vi "smsAt (SubVI).vi"() -> ()   [LabVIEW 2012]
doc: "Demonstrates general use of Obtain Queue, queues and the effects different settings have on queue behavior. It uses a queue to pass data between an Enqueue loop (producing data) and a Dequeue loop (consuming data). If both loops run at the same speed, the queue does not fill up.\n\nWhen the Enqueue loop runs fast and the Dequeue loop runs slow, the queue quickly fills up and the Enqueue loop must wait for the Dequeue loop to remove elements. If the Enqueue loop runs slow and the Dequeue loop runs fast, the queue is quickly emptied and the Dequeue loop must wait for the Enqueue loop to insert elements."
uses:
  <vilib>/Instr/_visa.llb/VISA Set IO Buffer Mask.ctl
  <vilib>/Instr/_visa.llb/VISA Configure Serial Port (Instr).vi
panel:
  out "num":string
  out "read buffer":string
  out "Serial Settings:Data Bits":u16
  in  "VISA resource name":refnum<visa-resource-name>="COM4"
  out "last SMS":string
  out "Elements in Queue":i32
  in  "stop":bool
  in  "Queue Size":i32=50
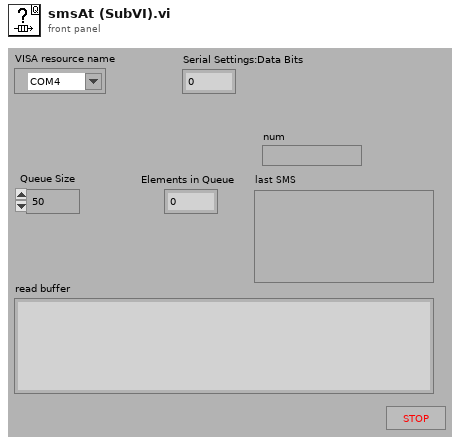
[diagram p1: front panel]
types:
  T1 = typedef "VISA Set IO Buffer Mask.ctl" = u16
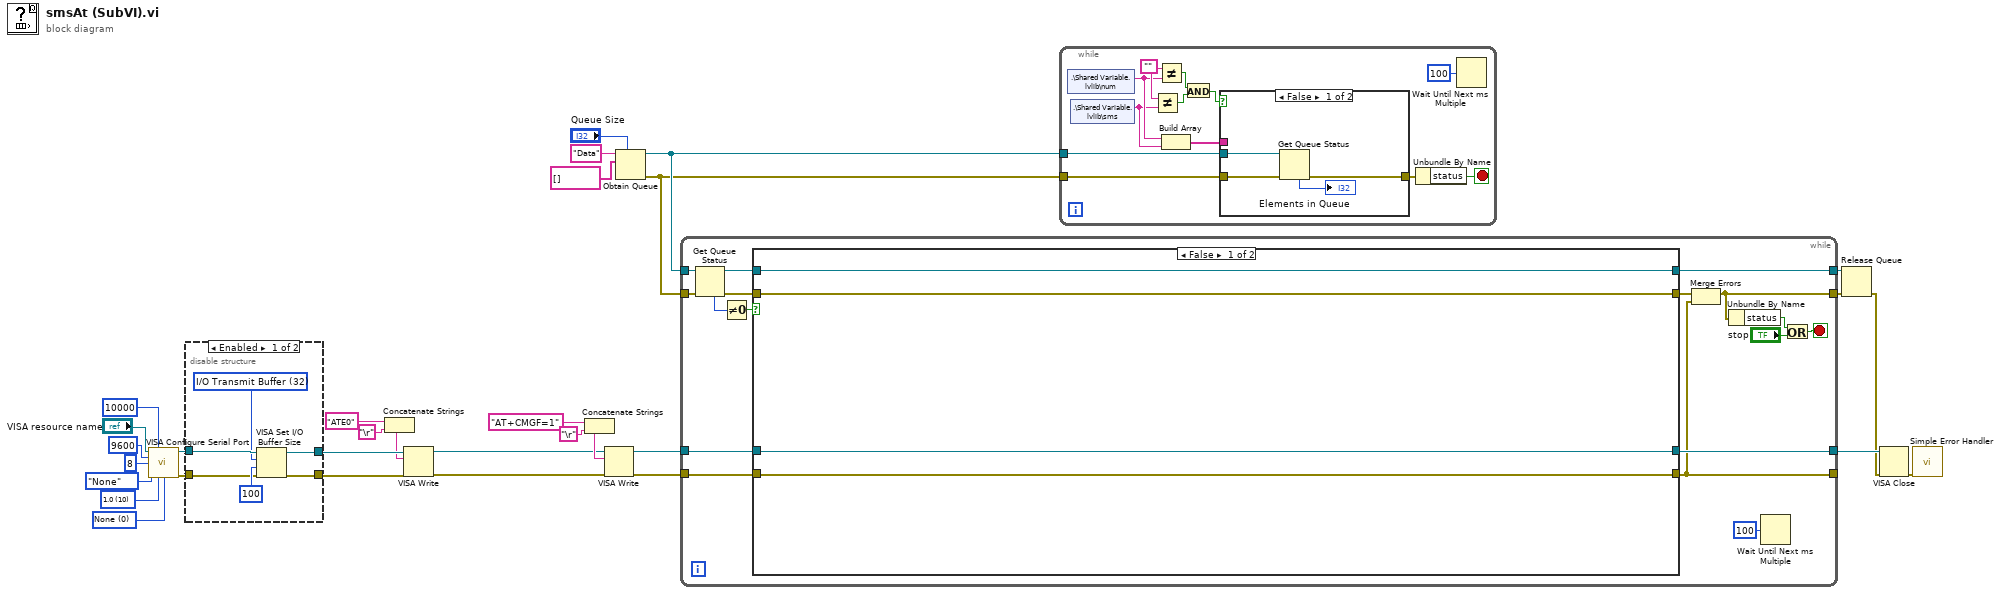
[diagram p0: block diagram]
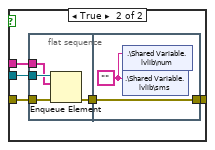
[diagram p3: hidden frame]
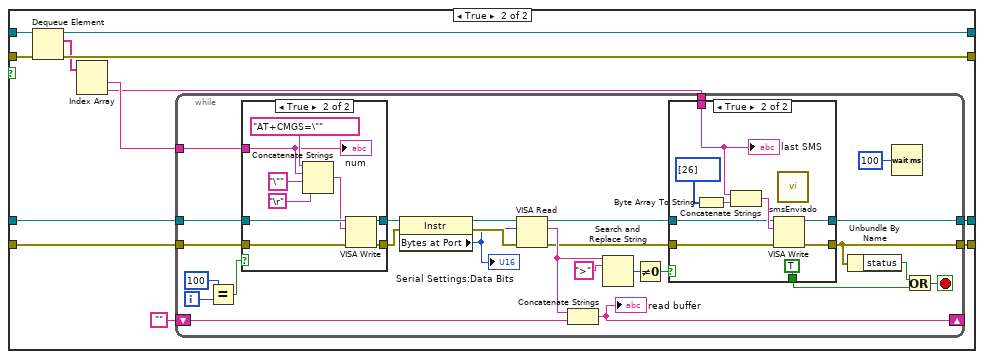
[diagram p4: hidden frame]
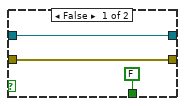
[diagram p5: hidden frame]
diagram:
  w22 = u16 0 items=["None", "XON/XOFF", "RTS/CTS", "XON/XOFF & RTS/CTS", "DTR/DSR", "XON/XOFF & DTR/DSR"] ("flow control (0:none)")
  w26 = u16 10 items=["1.0"=10, "1.5"=15, "2.0"=20] ("stop bits (10: 1 bit)")
  n1 = call-poly "VISA Configure Serial Port"("VISA resource name"="VISA resource name", "timeout (10sec)"=u32 10000, "baud rate (9600)"=u32 9600, "data bits (8)"=u16 8, "parity (0:none)"=enum16{"None", "Odd", "Even", "Mark", "Space"}."None", "stop bits (10: 1 bit)"=w26, "flow control (0:none)"=w22) -> ("VISA resource name out"=w20:refnum<visa-resource-name>, "error out"=w14:errorcluster)  [unwired: 7 in]
  n2 = disable-structure shown="Enabled" {
    disable-tunnel: w20 -> [w37 w39]
    disable-tunnel: [w34 w39] -> w19
    disable-tunnel: [w33 w38] -> w18
    disable-tunnel: w14 -> [w32 w38]
    frame Enabled {
      w35 = T1 32 items=["I/O Receive Buffer"=16, "I/O Transmit Buffer"=32, "I/O Receive and Transmit Buffer"=48] ("Mask")
      n3 = VISA Set I/O Buffer Size(VISA resource name=w37, mask (16)=w35, size (4096)=u32 100, error in (no error)=w32) -> (VISA resource name out=w34:refnum<visa-resource-name>, error out=w33:errorcluster)
    }
    frame Disabled {
    }
  }
  n4 = Concatenate Strings("ATE0" ("write buffer"), "\r") -> (w15:string)
  n5 = VISA Write(VISA resource name=w19, write buffer=w15, error in (no error)=w18) -> (VISA resource name out=w3:refnum<visa-resource-name>, error out=w4:errorcluster)  [unwired: 1 out]
  n6 = Concatenate Strings("AT+CMGF=1" ("write buffer"), "\r") -> (w7:string)
  n7 = VISA Write(VISA resource name=w3, write buffer=w7, error in (no error)=w4) -> (VISA resource name out=w2:refnum<visa-resource-name>, error out=w1:errorcluster)  [unwired: 1 out]
  n8 = Obtain Queue(max queue size (-1, unlimited)="Queue Size", name (unnamed)="Data", element data type=string[] []) -> (queue out=w31:refnum<queue>, error out=w29:errorcluster)  [unwired: 2 in, 1 out]
  n9 = while {
    tunnel: w31 -> [w56]
    tunnel: w29 -> [w52]
    tunnel: [w47] -> w28
    tunnel: w2 -> [w45]
    tunnel: w1 -> [w46]
    tunnel: [w44] -> w12
    tunnel: [w41] -> _
    tunnel: [w40] -> w10
    stop <- w55 stop-if-true
    n10 = Get Queue Status(queue=w56, error in (no error)=w52) -> (queue out=w48:refnum<queue>, error out=w49:errorcluster, # elements in queue=w51:i32)  [unwired: 6 out]
    n11 = Not Equal To 0?(x=w51) -> (x != 0?=w50:bool)
    n12 = case shown="False" w50 {
      tunnel: w49 -> [w59 w70]
      tunnel: [w59 w69] -> w42
      tunnel: w48 -> [w60 w72]
      tunnel: [w60 w71] -> w47
      tunnel: w46 -> [w57 w61]
      tunnel: w45 -> [w58 w62]
      tunnel: [w58 w67] -> w44
      tunnel: [w57 w66] -> w41
      frame False {
      }
      frame True {
        n13 = Dequeue Element(queue=w72, error in (no error)=w70) -> (queue out=w71:refnum<queue>, element=w65:string[], error out=w69:errorcluster)  [unwired: 2 out]
        n14 = Index Array(array=w65) -> (element #1=w64:string, element #2=w63:string)  [unwired: 2 in]
        n15 = while {
          tunnel: [w79] -> w66
          tunnel: [w86] -> w67
          shift-right: [w95] -> _
          shift-left: "" -> [w94]
          tunnel: w62 -> [w93]
          tunnel: w61 -> [w92]
          tunnel: w63 -> [w75]
          tunnel: w64 -> [w74]
          i -> [w81]
          stop <- w76 stop-if-true
          n16 = Equal?(x=100, y=w81) -> (x = y?=w80:bool)
          n17 = case shown="True" w80 {
            tunnel: [w112 w117] -> w97
            tunnel: [w111 w116] -> w96
            tunnel: w93 -> [w112 w119]
            tunnel: w92 -> [w111 w118]
            tunnel: w74 -> [_ w113]
            frame False {
            }
            frame True {
              n18 = Concatenate Strings("AT+CMGS=\"", w113, "\"" ("string"), "\r") -> (w115:string)
              n19 = VISA Write(VISA resource name=w119, write buffer=w115, error in (no error)=w118) -> (VISA resource name out=w117:refnum<visa-resource-name>, error out=w116:errorcluster)  [unwired: 1 out]
              "num" <- w113
            }
          }
          n20 = property class="Instr"(reference=w97, error in=w96) -> (reference out=w98:refnum<visa-resource-name>, error out=w84:errorcluster, "Bytes at Port"=w83:u32)
          "Serial Settings:Data Bits" <- w83
          n21 = VISA Read(VISA resource name=w98, byte count=w83, error in (no error)=w84) -> (VISA resource name out=w87:refnum<visa-resource-name>, read buffer=w91:string, error out=w85:errorcluster)  [unwired: 1 out]
          n22 = Concatenate Strings(w91, w94) -> (w95:string)
          "read buffer" <- w95
          n23 = Search and Replace String(input string=w91, search string=">") -> (number of replacements=w89:i32)  [unwired: 6 in, 3 out]
          n24 = Not Equal To 0?(x=w89) -> (x != 0?=w88:bool)
          n25 = case shown="True" w88 {
            tunnel: w87 -> [w101 w109]
            tunnel: [w101 w107] -> w86
            tunnel: w85 -> [w100 w108]
            tunnel: [w100 w106] -> w79
            tunnel: [FALSE TRUE] -> w77
            tunnel: w75 -> [_ w102]
            frame False {
            }
            frame True {
              n26 = Byte Array To String(unsigned byte array=u8[] [26]) -> (string=w104:string)
              n27 = Concatenate Strings(w102, w104) -> (w110:string)
              n28 = VISA Write(VISA resource name=w109, write buffer=w110, error in (no error)=w108) -> (VISA resource name out=w107:refnum<visa-resource-name>, error out=w106:errorcluster)  [unwired: 1 out]
              n29 = call "smsEnviado.vi"() -> ()  [unwired: 12 in]
              "last SMS" <- w102
            }
          }
          n30 = Unbundle By Name(w79) -> ("status"=w78:bool)
          n31 = Wait (ms)(milliseconds to wait=u32 100) -> ()  [unwired: 1 out]
          n32 = Or(x=w78, y=w77) -> (x .or. y?=w76:bool)
        }
      }
    }
    n33 = Merge Errors(w42, w41) -> (w40:errorcluster)
    n34 = Unbundle By Name(w40) -> ("status"=w54:bool)
    n35 = Wait Until Next ms Multiple(millisecond multiple=u32 100) -> ()  [unwired: 1 out]
    n36 = Or(x=w54, y="stop") -> (x .or. y?=w55:bool)
  }
  n37 = while {
    tunnel: w31 -> [w133]
    tunnel: w29 -> [w132]
    stop <- w129 stop-if-true
    w128 = ""
    n38 = shared-variable ".\\Shared Variable.lvlib\\num"() -> (w123:string)  [unwired: 1 in, 1 out]
    n39 = shared-variable ".\\Shared Variable.lvlib\\sms"() -> (w122:string)  [unwired: 1 in, 1 out]
    n40 = Not Equal?(x=w128, y=w122) -> (x != y?=w127:bool)
    n41 = Not Equal?(x=w128, y=w123) -> (x != y?=w126:bool)
    n42 = Build Array(w123, w122) -> (w125:string[])
    n43 = And(x=w126, y=w127) -> (x .and. y?=w124:bool)
    n44 = case shown="False" w124 {
      tunnel: w133 -> [w137 w142]
      tunnel: w132 -> [w136 w141]
      tunnel: [w135 w140] -> w130
      tunnel: w125 -> [_ w139]
      frame False {
        n45 = Get Queue Status(queue=w137, error in (no error)=w136) -> (error out=w135:errorcluster, # elements in queue=→"Elements in Queue":i32)  [unwired: 7 out]
      }
      frame True {
        n46 = flat-sequence {
          tunnel: w142 -> [w146]
          tunnel: w141 -> [w145]
          tunnel: w139 -> [w143]
          tunnel: [w144] -> w138
          tunnel: [w148] -> w140
          tunnel: w138 -> [w148]
          frame #0 {
            n47 = Enqueue Element(queue=w146, element=w143, error in (no error)=w145) -> (error out=w144:errorcluster)  [unwired: 3 out]
          }
          frame #1 {
            w147 = ""
            n48 = shared-variable ".\\Shared Variable.lvlib\\num"(w147) -> ()  [unwired: 1 in, 1 out]
            n49 = shared-variable ".\\Shared Variable.lvlib\\sms"(w147) -> ()  [unwired: 1 in, 1 out]
          }
        }
      }
    }
    n50 = Unbundle By Name(w130) -> ("status"=w129:bool)
    n51 = Wait Until Next ms Multiple(millisecond multiple=u32 100) -> ()  [unwired: 1 out]
  }
  n52 = Release Queue(queue=w28, error in (no error)=w10) -> (error out=w9:errorcluster)  [unwired: 3 out]
  n53 = VISA Close(VISA resource name=w12, error in (no error)=w9) -> (error out=w8:errorcluster)
  n54 = call <vilib>:"Simple Error Handler.vi"("error in (no error)"=w8) -> ()  [unwired: 1 in, 8 out]
